vi "Read Obs Time.vi"(8 "error in (no error)":errorcluster, 11 "Check Ozone Stability in":refnum<class "Check Ozone Stability.lvclass">) -> (0 "error out":errorcluster, 2 "Obs Time":dbl, 3 "Check Ozone Stability out":refnum<class "Check Ozone Stability.lvclass">)   [LabVIEW 2012, in "Check Ozone Stability.lvclass"]
uses:
  Check Ozone Stability.lvclass
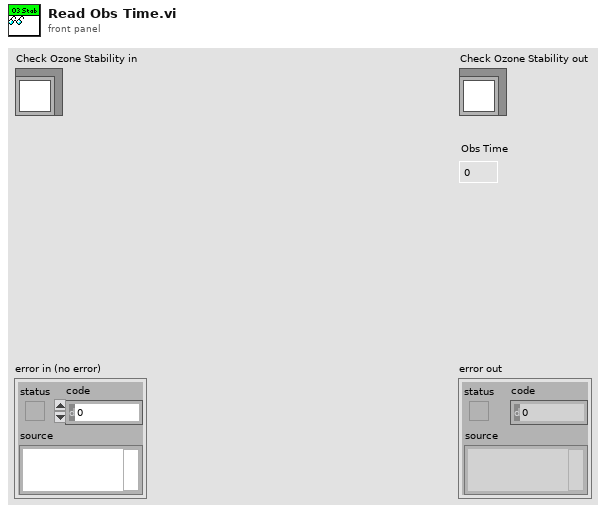
[diagram p1: front panel]
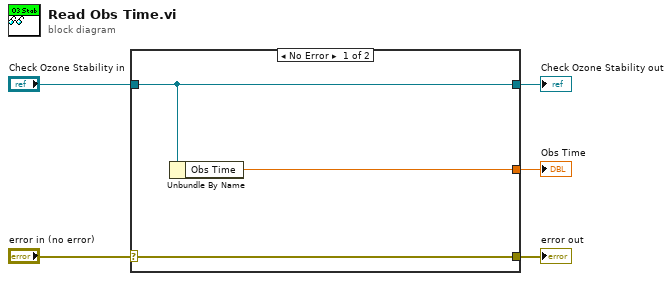
[diagram p0: block diagram]
diagram:
  n1 = case shown="No Error" "error in (no error)" {
    selector: "error in (no error)" -> [w8 w9]
    tunnel: [w8 w9] -> w4
    tunnel: [w7 w10] -> w2
    tunnel: "Check Ozone Stability in" -> [w7 w10]
    tunnel: [w6 _] -> w1
    frame No Error {
      n2 = Unbundle By Name(w7) -> ("Obs Time"=w6:dbl)
    }
    frame Error {
    }
  }
  "error out" <- w4
  "Check Ozone Stability out" <- w2
  "Obs Time" <- w1
